vi "WaveformSplitOnTimeBase.vi"(0 "Waveform In":waveform(dbl)={"t0"=timestamp(287278225.734 s since 1904-01-01), "dt"=0.0, "Y"=[], "attributes"=variant("Name"=variant(string "FringeTracker[0].CompleteControllerSet.ControllerData.ChannelData[0].CalibratedBinData[0]"))}, 1 "dt":dbl) -> (2 "Residual Before":waveform(dbl), 3 "Waveform Array":waveform(dbl)[](array[waveform]), 4 "Residual After":waveform(dbl)={"t0"=timestamp(287278225.734 s since 1904-01-01), "dt"=0.0, "Y"=[], "attributes"=variant("Name"=variant(string "FringeTracker[0].CompleteControllerSet.ControllerData.ChannelData[0].CalibratedBinData[0]"))})   [LabVIEW 2009]
uses:
  <vilib>/Waveform/WDTOps.llb/WDT Get Final Time Value DBL.vi
  <vilib>/Waveform/WDTOps.llb/WDT Waveform Duration DBL.vi
panel:
  out "tStop":dbl=48625.734 format="%.6g"
  out "size(s)":i32
  out "tStart":dbl=48625.734 format="%.6g"
  out "tSplit":dbl=nan format="%.6g"
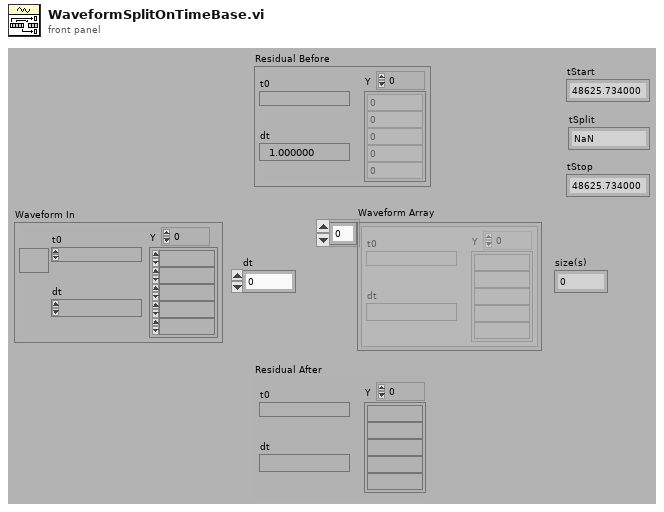
[diagram p1: front panel]
types:
  T1 = typedef "LVDateTimeRec.ctl" = cluster{"fractional second":dbl, "second":i32, "minute":i32, "hour":i32, "day of month":i32, "month":i32, "year":i32, "day of week":i32, "day of year":i32, "DST":i32}
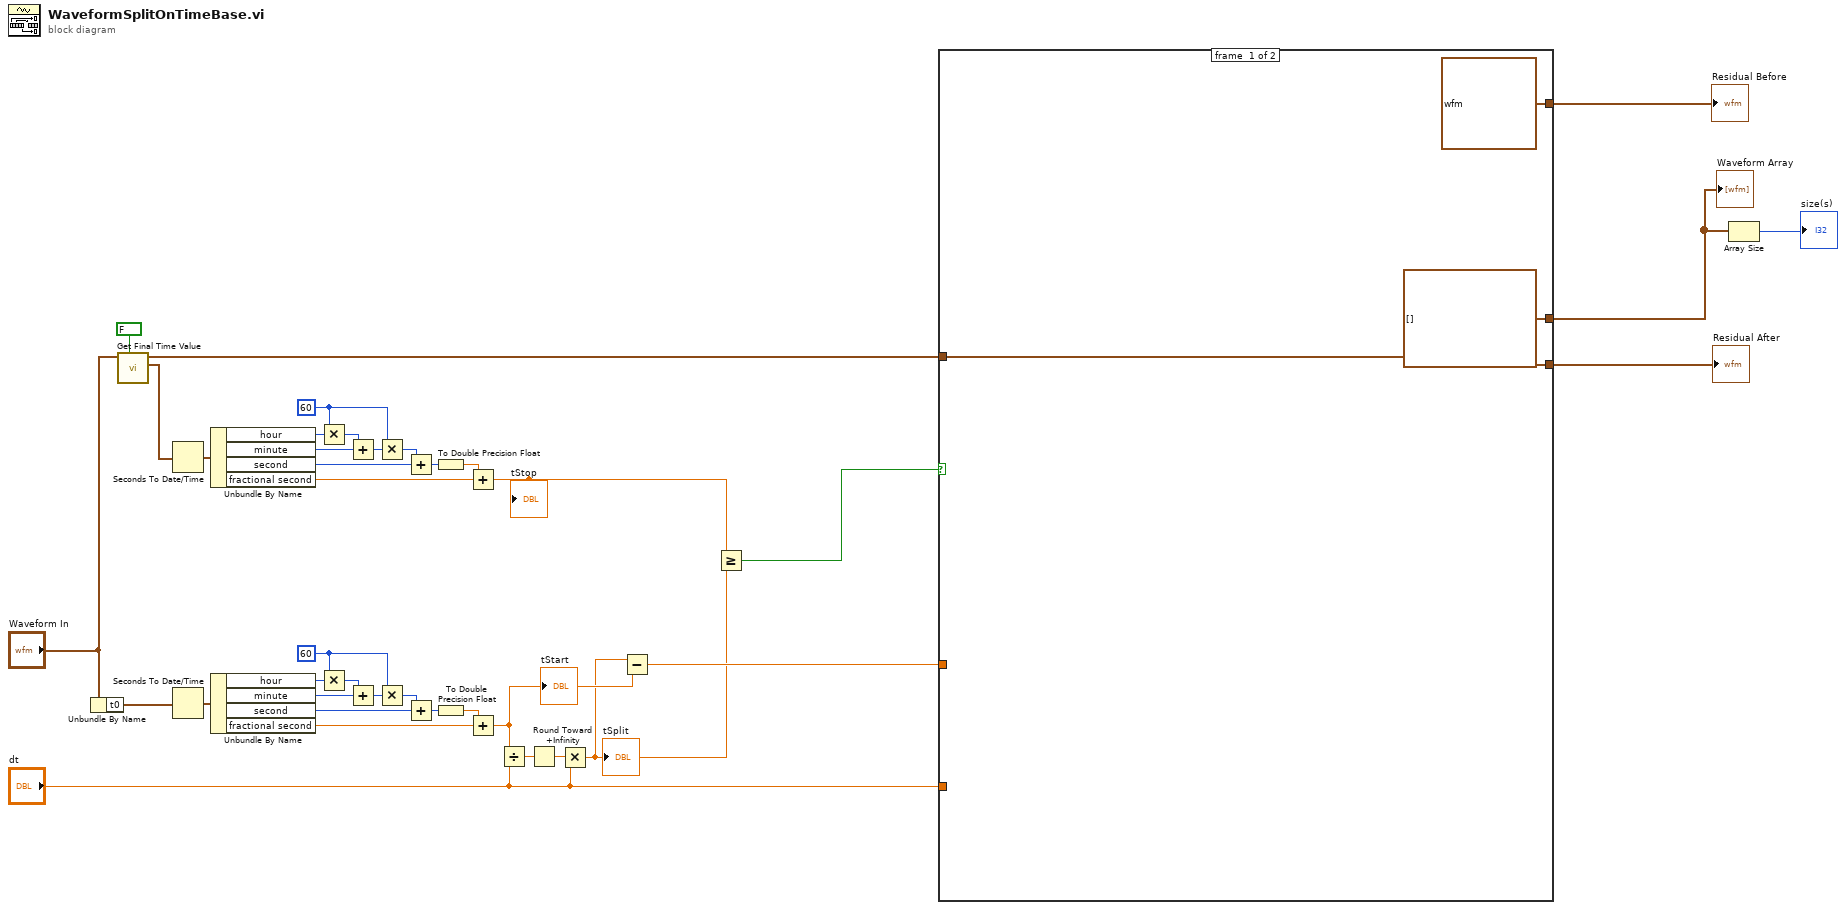
[diagram p0: block diagram]
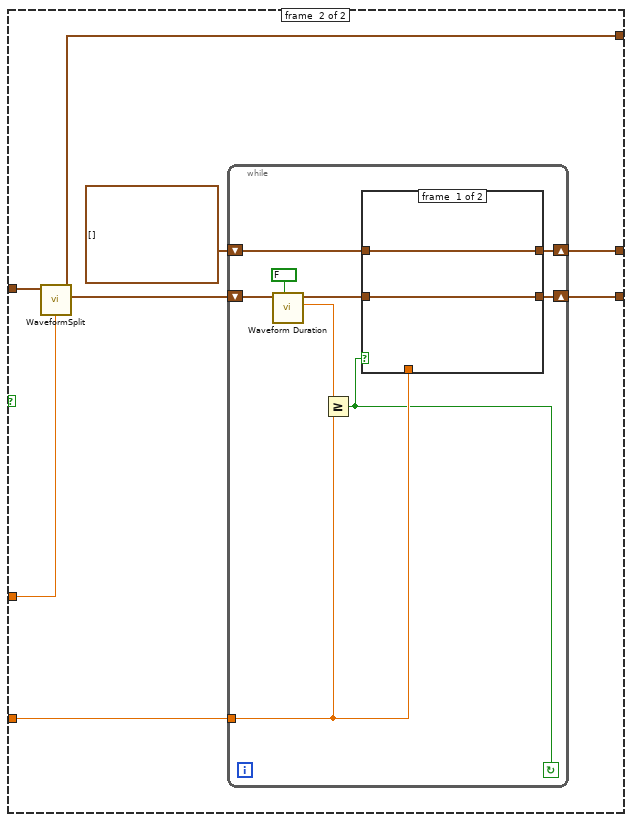
[diagram p2: hidden frame]
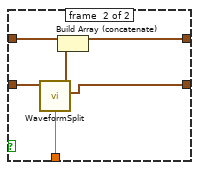
[diagram p3: hidden frame]
diagram:
  w11 = 60 ("x")
  w33 = 60 ("x")
  n1 = Unbundle By Name("Waveform In") -> ("t0"=w39:timestamp)
  n2 = call-poly <vilib>:"Get Final Time Value.vi"("open interval? (T)"=FALSE, "waveform in"="Waveform In") -> ("tf"=w5:timestamp, "waveform out"=w18:waveform(dbl))  [unwired: 1 in, 7 out]
  n3 = Seconds To Date/Time(time stamp (now)=w5) -> (date time rec=w6:T1)  [unwired: 1 out]
  n4 = Seconds To Date/Time(time stamp (now)=w39) -> (date time rec=w38:T1)  [unwired: 1 out]
  n5 = Unbundle By Name(w6) -> ("hour"=w7:i32, "minute"=w9:i32, "second"=w12:i32, "fractional second"=w15:dbl)
  n6 = Unbundle By Name(w38) -> ("hour"=w37:i32, "minute"=w35:i32, "second"=w32:i32, "fractional second"=w29:dbl)
  n7 = Multiply(x=w11, y=w7) -> (x*y=w8:i32)
  n8 = Multiply(x=w33, y=w37) -> (x*y=w36:i32)
  n9 = Add(x=w8, y=w9) -> (x+y=w10:i32)
  n10 = Add(x=w36, y=w35) -> (x+y=w34:i32)
  n11 = Multiply(x=w11, y=w10) -> (x*y=w13:i32)
  n12 = Multiply(x=w33, y=w34) -> (x*y=w31:i32)
  n13 = Add(x=w13, y=w12) -> (x+y=w14:i32)
  n14 = Add(x=w31, y=w32) -> (x+y=w30:i32)
  n15 = To Double Precision Float(number=w14) -> (double precision float=w16:dbl)
  n16 = To Double Precision Float(number=w30) -> (double precision float=w28:dbl)
  n17 = Add(x=w16, y=w15) -> (x+y=w4:dbl)
  "tStop" <- w4
  n18 = Add(x=w28, y=w29) -> (x+y=w25:dbl)
  "tStart" <- w25
  n19 = Divide(x=w25, y="dt") -> (x/y=w27:dbl)
  n20 = Round Toward +Infinity(x=w27) -> (ceil(x): smallest int >= x=w26:dbl)
  n21 = Multiply(x=w26, y="dt") -> (x*y=w3:dbl)
  "tSplit" <- w3
  n22 = Subtract(x=w3, y=w25) -> (x-y=w24:dbl)
  n23 = Greater Or Equal?(x=w4, y=w3) -> (x >= y?=w1:bool)
  n24 = case shown="True" w1 {
    tunnel: w24 -> [_ w50]
    tunnel: "dt" -> [_ w48]
    tunnel: [w42 w46] -> w22
    tunnel: [waveform(dbl)[] [] w45] -> w21
    tunnel: w18 -> [w42 w44]
    tunnel: [waveform(dbl) {"t0"=timestamp(0 s since 1904-01-01), "dt"=1.0, "Y"=[]} ("A") w43] -> w2
    frame #0 {
    }
    frame #1 {
      n25 = call "WaveformSplit.vi"("signal in"=w44, "Duration"=w50) -> ("A"=w43:waveform(dbl), "B"=w49:waveform(dbl))  [unwired: 1 in, 5 out]
      n26 = while {
        tunnel: w48 -> [w56]
        shift-right: [w54] -> w45
        shift-left: waveform(dbl)[] [] -> [w55]
        shift-right: [w53] -> w46
        shift-left: w49 -> [w59]
        stop <- w52 continue-if-true
        n27 = call-poly <vilib>:"Waveform Duration.vi"("open interval? (T)"=FALSE, "waveform in"=w59) -> ("duration"=w58:dbl, "waveform out"=w57:waveform(dbl))  [unwired: 1 in, 7 out]
        n28 = Greater Or Equal?(x=w58, y=w56) -> (x >= y?=w52:bool)
        n29 = case shown="True" w52 {
          tunnel: w57 -> [w61 w67]
          tunnel: w56 -> [_ w66]
          tunnel: w55 -> [w60 w65]
          tunnel: [w60 w63] -> w54
          tunnel: [w61 w62] -> w53
          frame #0 {
          }
          frame #1 {
            n30 = call "WaveformSplit.vi"("signal in"=w67, "Duration"=w66) -> ("A"=w64:waveform(dbl), "B"=w62:waveform(dbl))  [unwired: 1 in, 5 out]
            n31 = Build Array (concatenate)(w65, w64) -> (w63:waveform(dbl)[])
          }
        }
      }
    }
  }
  "Residual Before" <- w2
  "Waveform Array" <- w21
  "Residual After" <- w22
  n32 = Array Size(array=w21) -> (size(s)=→"size(s)":i32)
